vi "Pelletron_Controller.vi"() -> ()   [LabVIEW 2012, in "AccelNET.lvlib" / "Control_VIs.lvlib"]
uses:
  Control_VIs.lvlib
  Component_Power_Indicator.ctl
  Interlocks.ctl
  Bypass_Indicator.ctl
  Parameters_Indicator.ctl
  Parameters_Control.ctl
  Conditioning.ctl
  Component_Power_Control.ctl
  Bypass_Control.ctl
  Database2.0/Public API/PelletronLabview.ctl
  <vilib>/Utility/miscctls.llb/LVPointTypeDef.ctl
  TCPinfo.vi
  TCP.lvclass
  Global_Variables.lvlib
  Useful_SubVIs.lvlib
  Useful_Controls.lvlib
panel:
  out "uA/kV":dbl
  in  "Post to database?":bool=TRUE
  out "Connection Status":bool
  out "Bypass Turn Off":dbl format="%<%H:%M:%S>t"
  in  "Synch":bool
  out "Interlock Status":T1
  in  "Y Log Scale?":bool
  in  "X Maximum":dbl max=0.0 step=30.0 format="%<%H:%M:%S>t"
  in  "X Autoscale":bool=TRUE
  in  "X Minimum":dbl max=0.0 step=30.0 format="%<%H:%M:%S>t"
  in  "Y Autoscale":bool=TRUE
  in  "Y Maximum":dbl
  in  "Y Minimum":dbl
  out "Start Time":dbl format="%<%m/%d/%Y  -  %H:%M:%S>T"
  in  "Clear":bool
  out "XY Graph":cluster{dbl[], dbl[]}(graph)
  in  "Plotter Selector":u16(ring) items=["High Voltage", "High Voltage PS", "Chain Current", "Column Current", "Lost Charge", "Radiation", "Pressure", "HV Control Difference"]
  out "Stop Checking for Sparks Start":dbl
  in  "Stop Condition":bool
  in  "Spark Counter Reset":bool
  in  "Update Parameters":bool
  in  "Param Controls":T2 {"Control Reference\nVoltage (MV)" min=0.3 max=3.0 step=0.1; "High Voltage\nPS Setting (kV)" min=0.0 max=18.0 step=0.2; "Spark\nLimit" min=0.0 max=10.0 step=1.0}
  out "Parameters":T3 {"High\nVoltage (MV)" format="%#.4g"; "Control Reference\nVoltage (MV)" format="%#.4g"; "+ High Voltage\nPS (kV)" format="%#.4g"; "- High Voltage\nPS (kV)" format="%#.4g"; "HV Control\nDifference (kV)" format="%#.4g"; "High Voltage\nPS Setting (kV)" format="%#.4g"; "Chain\nCurrent (uA)" format="%#.4g"; "Column\nCurrent (uA)" format="%#.4g"; "Spark\nLimit" format="%#.0g"; "Spark\nCount" format="%#.0g"; "Lost Charge (uA)" scale=-10.0..10.0; "Spark\nThreshold (MV)" format="%#.4g"; "Radiation (mRad/hr)" step=3.978696e-316 scale=0.02..200.0 scale format="%#.4f"; "Vacuum (Torr)" scale=1e-09..0.001 scale format="%#_6e"}
  out "Warning!":bool
  in  "Reset":bool
  out "Rad. Avg.":dbl(slide) scale=0.02..200.0 scale format="%.0e"
  out "Stopped":bool
  out "Spark\nCounter":i64
  in  "Spark Limit":i64=2
  in  "Emergency Stop":bool
  out "Accelnet Write Errors":errorcluster
  in  "Clear Errors":bool
  out "Accelnet Read Errors":errorcluster
  in  "stop":bool
  out "Condition\nStart Time":dbl format="%<%H:%M:%S>T"
  in  "Conditioning":T4
  in  "Bypass Control":T5
  in  "Update Bypass":bool
  out "Pelletron Bypass":T6
  in  "Component Power Control":T7
  in  "Update On/off":bool
  out "Component\nPower":T8
  # "Instructions:\n\n1) Make sure TCP Control is on and the connection is open.  This is true if you can see TCP information on the top where it says IP Address.\n\n2) Turn on the Pelletron Controller\n\n3) Check to see that the Blower and Ion Gauge Filament is on\n\n4) Check all interlocks are lighte and all bypasses are not.\n\n5) Controls are separate from readings.  Pressing the update button in each respective section sends the commands to the Accelnet system.\n\n6) If the Stopped light is on, then the system will lock out all Pelletron controls and shut off the system until the Reset button is pressed.\n\n7) When finished, stop program with Stop button (make sure Pelletron is off)."
  # "Pelletron Startup Sequence:\n1.  Turn on HV Power Supply\n2. Check +High Voltage PS under parameters to be 1 kV if not change it using the High Voltage PS Setting\n3. Turn on Chain PS\n4. Turn on Chain\n5. Condition Pelletron using auto conditioner or manually using High Voltage PS Setting under Parameter Control\n6.  Check Control Reference Voltage under Parameters to be desired voltage and change it if it is not\n7.  Open Beamline Gate Valve\n8.  Turn on Control Mode\n9.  Turn on Rotating Shaft\n10. Operate Pelletron source through Andrew's Box"
  # "Pelletron Shutdown Sequence:\n1.  Make sure Andrew's box is turned down and off\n2.  Turn off Rotating Shaft\n3.  Check High Voltage PS Setting to be close to + High Voltage PS, if not set it to ~0.2kV above the current setting\n4.  Turn off Control Mode\n5. Close Beamline Gatevalve\n         a.  If you are leaving the pelletron on but the accelerator off, stop here.\n6.  Set Voltage to 1 kv using HighVoltage PS Setting\n7.  Turn off Chain\n8.  Turn off Chain PS and HV Power Supply\n9.  Stop the program."
  # "Interlocks"
  # "Pelletron Plotter"
  # "Parameter Control"
  # "Parameters"
  # "LabVIEW Interlocks"
  # "Pelletron\n   Stop"
  # "Conditioning"
  # "Bypass"
  # "Component On/Off"
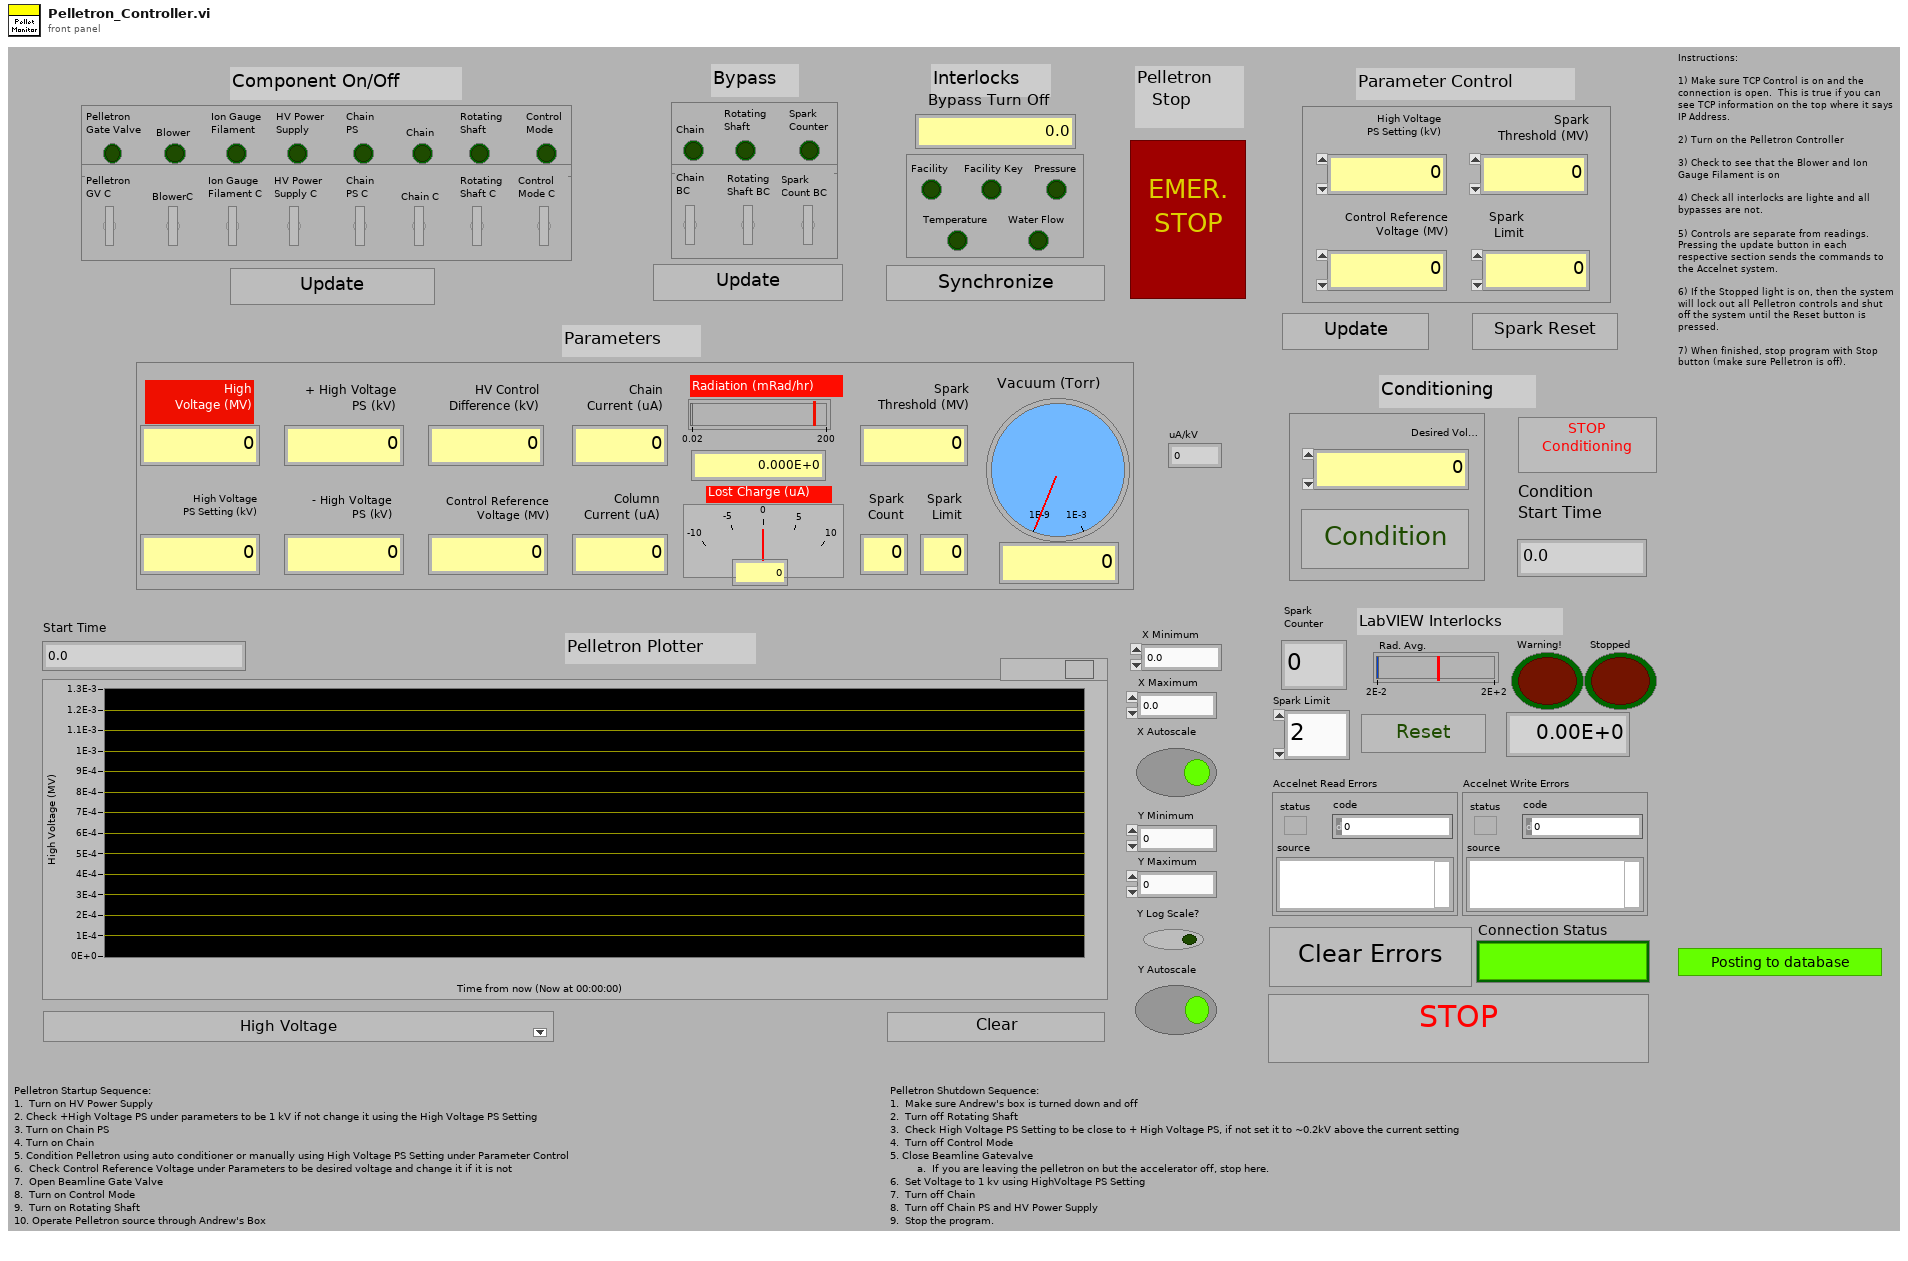
[diagram p1: front panel]
types:
  T1 = typedef "AccelNET.lvlib/Useful_Controls.lvlib/Interlocks.ctl" = cluster{"Facility":bool, "Facility Key":bool, "Water Flow":bool, "Pressure":bool, "Temperature":bool}
  T2 = typedef "AccelNET.lvlib/Useful_Controls.lvlib/Parameters_Control.ctl" = cluster{"Spark\nThreshold (MV)":dbl, "Spark\nLimit":dbl, "High Voltage\nPS Setting (kV)":dbl, "Control Reference\nVoltage (MV)":dbl}
  T3 = typedef "AccelNET.lvlib/Useful_Controls.lvlib/Parameters_Indicator.ctl" = cluster{"Vacuum (Torr)":dbl, "Radiation (mRad/hr)":dbl, "Spark\nThreshold (MV)":dbl, "Lost Charge (uA)":dbl, "Spark\nCount":dbl, "Spark\nLimit":dbl, "Column\nCurrent (uA)":dbl, "Chain\nCurrent (uA)":dbl, "High Voltage\nPS Setting (kV)":dbl, "HV Control\nDifference (kV)":dbl, "- High Voltage\nPS (kV)":dbl, "+ High Voltage\nPS (kV)":dbl, "Control Reference\nVoltage (MV)":dbl, "High\nVoltage (MV)":dbl}
  T4 = typedef "AccelNET.lvlib/Useful_Controls.lvlib/Conditioning.ctl" = cluster{"Desired Voltage (MV)":dbl, "Conditioning?":bool}
  T5 = typedef "AccelNET.lvlib/Useful_Controls.lvlib/Bypass_Control.ctl" = cluster{"Chain\nBC":bool, "Rotating\nShaft BC":bool, "Spark\nCount BC":bool}
  T6 = typedef "AccelNET.lvlib/Useful_Controls.lvlib/Bypass_Indicator.ctl" = cluster{"Chain":bool, "Rotating\nShaft":bool, "Spark\nCounter":bool}
  T7 = typedef "AccelNET.lvlib/Useful_Controls.lvlib/Component_Power_Control.ctl" = cluster{"Pelletron\nGV C":bool, "BlowerC":bool, "Chain C":bool, "Rotating\nShaft C":bool, "HV Power\nSupply C":bool, "Ion Gauge\nFilament C":bool, "Control\nMode C":bool, "Chain\nPS C":bool}
  T8 = typedef "AccelNET.lvlib/Useful_Controls.lvlib/Component_Power_Indicator.ctl" = cluster{"Pelletron\nGate Valve":bool, "Blower":bool, "Chain":bool, "Rotating\nShaft":bool, "HV Power\nSupply":bool, "Ion Gauge\nFilament":bool, "Control\nMode":bool, "Chain\nPS":bool}
  T9 = typedef "LVPointTypeDef.ctl" = cluster{"Horizontal":i16, "Vertical":i16}
  T10 = typedef "PelletronLabview.ctl" = cluster{"Timestamp":timestamp, "High Voltage":sgl, "+ High Voltage Supply":dbl, "- High Voltage Supply":dbl, "HV Control Difference":dbl, "Vacuum Pressure":sgl, "Radiation":dbl, "Column Current":sgl, "Lost Charge":dbl, "Chain Current":sgl, "Control High Voltage":dbl}
  T11 = cluster{"Time":dbl, "High Voltage":dbl, "High VoltagePS":dbl, "Chain Current":dbl, "Column Current":dbl, "Lost Charge":dbl, "Radiation":dbl, "Pressure":dbl, "HV Control Difference":dbl}[]
  T12 = cluster{"Spark\nThreshold (MV)":dbl, "Spark\nLimit":dbl, "High Voltage\nPS Setting (kV)":dbl, "Control Reference\nVoltage (MV)":dbl}
  T13 = enum8{"Enabled", "Disabled", "Disabled and Grayed Out"}
  T14 = cluster{"Time":dbl, "High Voltage":dbl, "High VoltagePS":dbl, "Chain Current":dbl, "Column Current":dbl, "Lost Charge":dbl, "Radiation":dbl, "Pressure":dbl, "HV Control Difference":dbl}
  T15 = cluster{"High\nVoltage (MV)":dbl, "Vacuum (Torr)":dbl, "Lost Charge (uA)":dbl, "+ High Voltage\nPS (kV)":dbl}
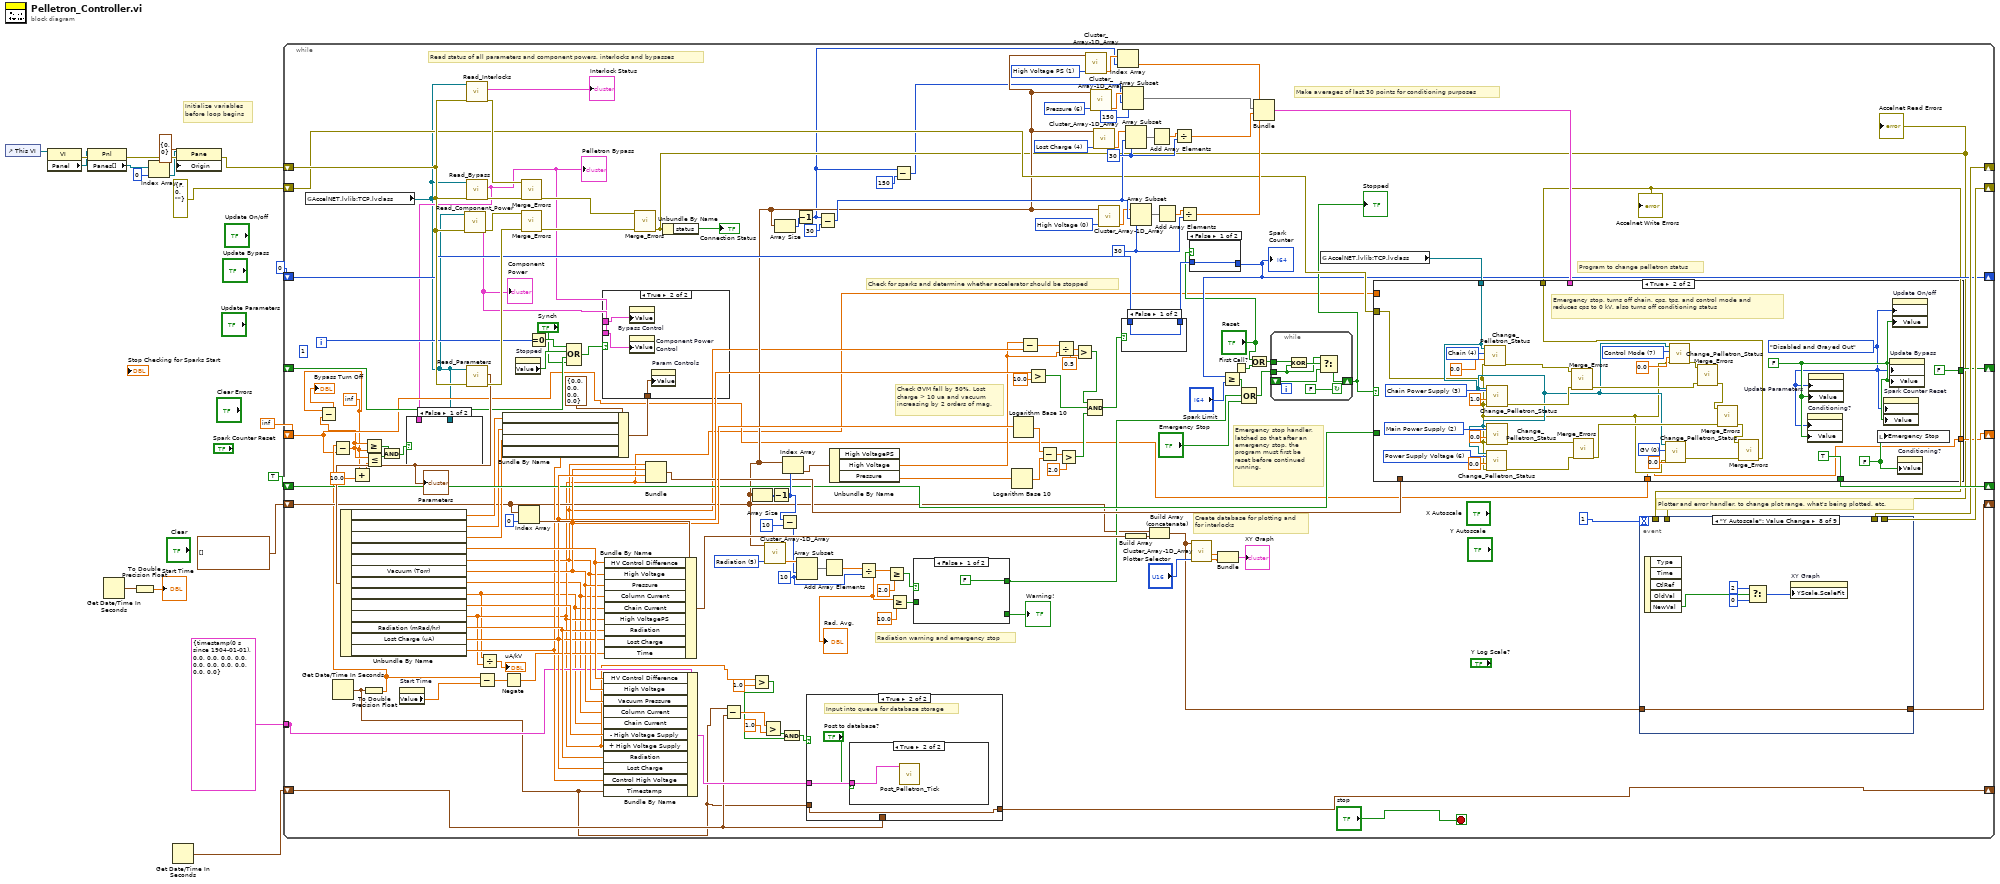
[diagram p0: block diagram]
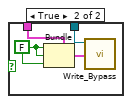
[diagram p4: hidden frame]
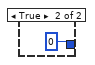
[diagram p5: hidden frame]
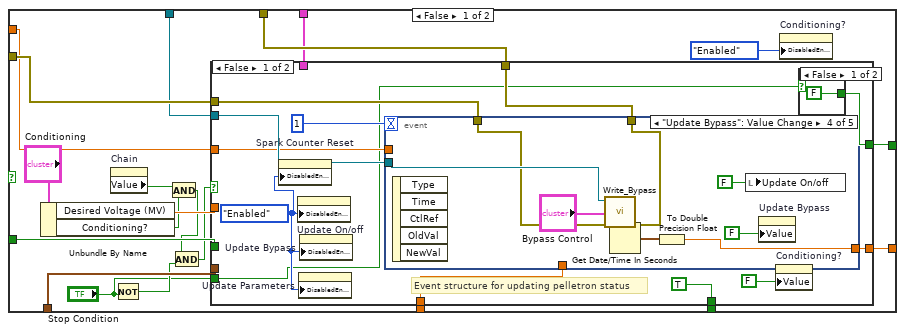
[diagram p7: hidden frame]
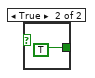
[diagram p8: hidden frame]
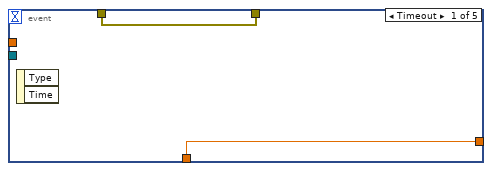
[diagram p9: hidden frame]
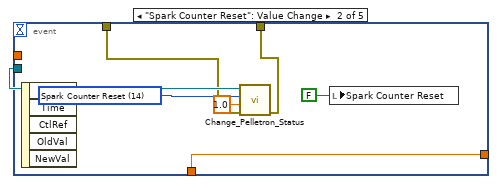
[diagram p10: hidden frame]
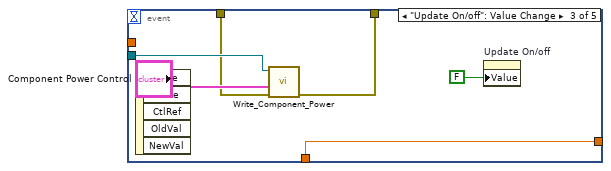
[diagram p11: hidden frame]
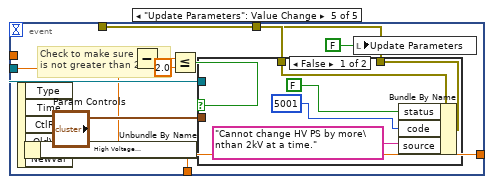
[diagram p12: hidden frame]
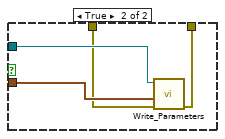
[diagram p13: hidden frame]
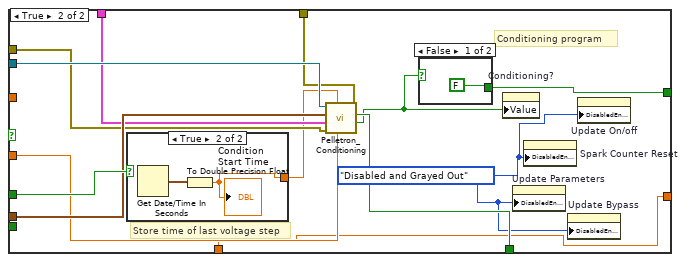
[diagram p14: hidden frame]
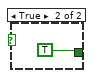
[diagram p15: hidden frame]
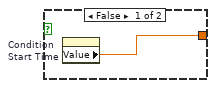
[diagram p16: hidden frame]
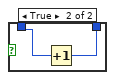
[diagram p17: hidden frame]
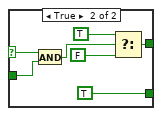
[diagram p18: hidden frame]
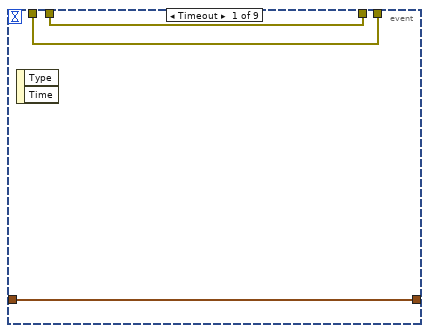
[diagram p19: hidden frame]
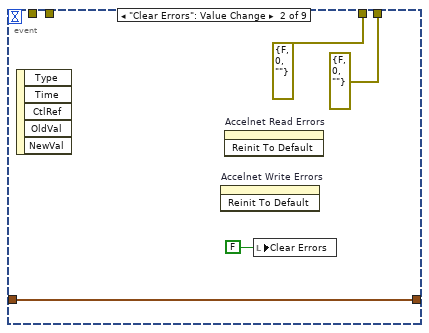
[diagram p20: hidden frame]
diagram:
  # "Initialize variables\nbefore loop begins"
  n1 = control-ref of="This VI"() -> (w9:refnum<vi>)
  n2 = property class="VI"(reference=w9) -> (error out=w8:errorcluster, "Panel"=w7:refnum<vi>)  [unwired: 1 in, 1 out]
  n3 = property class="Pnl"(reference=w7, error in=w8) -> (error out=w6:errorcluster, "Panes[]"=w5:refnum<vi>[])  [unwired: 1 out]
  n4 = Get Date/Time In Seconds() -> (seconds since 1Jan1904=w17:timestamp)
  n5 = To Double Precision Float(number=w17) -> (double precision float=→"Start Time":dbl)
  n6 = Index Array(array=w5, index=0) -> (element=w3:refnum<vi>)
  n7 = Get Date/Time In Seconds() -> (seconds since 1Jan1904=w10:timestamp)
  n8 = property class="Pane"(reference=w3, error in=w6, "Origin"=T9 {"Horizontal"=0, "Vertical"=0}) -> (error out=w1:errorcluster)  [unwired: 1 out]
  n9 = while {
    shift-right: [w98] -> _
    shift-left: w1 -> [w169]
    shift-right: [w154] -> _
    shift-left: T11 [] -> [w82]
    shift-right: [w79] -> _
    shift-left: i64 0 -> [w129]
    shift-right: [w97] -> _
    shift-left: errorcluster {"status"=FALSE, "code"=0, "source"=""} ("error out") -> [w87]
    shift-right: [w102] -> _
    shift-left: TRUE -> [w103]
    shift-right: [w56] -> _
    shift-left: _ -> [w55]
    shift-right: [w53] -> _
    shift-left: inf -> [w51]
    tunnel: [w33] -> _
    tunnel: T10 {"Timestamp"=timestamp(0 s since 1904-01-01), "High Voltage"=0.0, "+ High Voltage Supply"=0.0, "- High Voltage Supply"=0.0, "HV Control Difference"=0.0, "Vacuum Pressure"=0.0, "Radiation"=0.0, "Column Current"=0.0, "Lost Charge"=0.0, "Chain Current"=0.0, "Control High Voltage"=0.0} ("Cluster") -> [w33]
    shift-right: [w31] -> _
    shift-left: w10 -> [w28]
    i -> [w96]
    stop <- "stop" stop-if-true
    w38 = inf ("y")
    (unwired) 1
    w105 = u16 1 items=["High Voltage", "High Voltage PS", "Chain Current", "Column Current", "Lost Charge", "Radiation", "Pressure", "HV Control Difference"] ("Plotter Selector")
    w114 = u16 6 items=["High Voltage", "High Voltage PS", "Chain Current", "Column Current", "Lost Charge", "Radiation", "Pressure", "HV Control Difference"] ("Plotter Selector")
    w115 = 30 ("length")
    w118 = u16 4 items=["High Voltage", "High Voltage PS", "Chain Current", "Column Current", "Lost Charge", "Radiation", "Pressure", "HV Control Difference"] ("Plotter Selector")
    w121 = 30 ("length")
    w126 = u16 0 items=["High Voltage", "High Voltage PS", "Chain Current", "Column Current", "Lost Charge", "Radiation", "Pressure", "HV Control Difference"] ("Plotter Selector")
    w125 = 10 ("length")
    w142 = u16 5 items=["High Voltage", "High Voltage PS", "Chain Current", "Column Current", "Lost Charge", "Radiation", "Pressure", "HV Control Difference"] ("Plotter Selector")
    # "Emergency stop handler,\nlatched so that after an\nemergency stop, the \nprogram must first be \nreset before continued\nrunning."
    # "Plotter and error handler, to change plot range, what's being plotted, etc."
    # "Program to change pelletron status"
    # "Make averages of last 30 points for conditioning purposes"
    # "Check GVM fall by 50%, Lost\ncharge > 10 ua and vacuum\nincreasing by 2 orders of mag."
    # "Create database for plotting and\nfor interlocks"
    # "Radiation warning and emergency stop"
    # "Check for sparks and determine whether accelerator should be stopped"
    # "Read status of all parameters and component powers, interlocks and bypasses"
    n10 = global read "TCPinfo.vi" "AccelNET.lvlib:TCP.lvclass"() -> (w47:refnum<class "TCP.lvclass">)
    n11 = Get Date/Time In Seconds() -> (seconds since 1Jan1904=w27:timestamp)
    n12 = Add(x=w38, y=10.0) -> (x+y=w40:dbl)
    n13 = To Double Precision Float(number=w27) -> (double precision float=w52:dbl)
    n14 = Subtract(x=w52, y=w51) -> (x-y=w45:dbl)
    n15 = Subtract(x=w38, y=w45) -> (x-y=→"Bypass Turn Off":dbl)
    n16 = Greater Or Equal?(x=w45, y=w38) -> (x >= y?=w50:bool)
    n17 = Less Or Equal?(x=w45, y=w40) -> (x <= y?=w49:bool)
    n18 = And(x=w50, y=w49) -> (x .and. y?=w41:bool)
    n19 = property on="Start Time" class="DigNum (strict)"() -> ("Value"=w162:dbl)  [unwired: 2 in, 2 out]
    n20 = call "Read_Component_Power.vi"("error in (no error)"=w169, "AccelNET.lvlib:TCP.lvclass"=w47) -> ("Error Out"=w166:errorcluster, "Component Power"=w54:T8)  [unwired: 8 in]
    "Component\nPower" <- w54
    n21 = call "Read_Interlocks.vi"("Error In"=w169, "AccelNET.lvlib:TCP.lvclass"=w47) -> ("Error Out"=w168:errorcluster, "Interlock Status"=→"Interlock Status":T1)  [unwired: 8 in]
    n22 = call "Read_Bypass.vi"("error in (no error)"=w169, "AccelNET.lvlib:TCP.lvclass"=w47) -> ("Error Out"=w167:errorcluster, "Pelletron Bypass"=w48:T6)  [unwired: 8 in]
    "Pelletron Bypass" <- w48
    n23 = case shown="False" w41 {
      tunnel: w48 -> [_ w178]
      tunnel: w47 -> [_ w175]
      frame False {
      }
      frame True {
        w177 = FALSE ("Chain")
        n24 = Bundle(cluster=w178, "Chain"=w177, "Rotating\nShaft"=w177, "Spark\nCounter"=w177) -> (w176:T6)
        n25 = call "Write_Bypass.vi"("AccelNET.lvlib:TCP.lvclass"=w175, "Pelletron Bypass"=w176) -> ()  [unwired: 8 in, 1 out]
      }
    }
    n26 = call "Read_Parameters.vi"("error in (no error)"=w169, "AccelNET.lvlib:TCP.lvclass"=w47) -> ("Error Out"=w165:errorcluster, "Parameters"=w160:T3)  [unwired: 8 in]
    "Parameters" <- w160
    n27 = Unbundle By Name(w160) -> ("Spark\nThreshold (MV)"=w89:dbl, "Spark\nLimit"=w90:dbl, "High Voltage\nPS Setting (kV)"=w91:dbl, "HV Control\nDifference (kV)"=w147:dbl, "High\nVoltage (MV)"=w66:dbl, "Vacuum (Torr)"=w107:dbl, "Column\nCurrent (uA)"=w20:dbl, "Chain\nCurrent (uA)"=w19:dbl, "- High Voltage\nPS (kV)"=w148:dbl, "+ High Voltage\nPS (kV)"=w22:dbl, "Radiation (mRad/hr)"=w146:dbl, "Lost Charge (uA)"=w108:dbl, "Control Reference\nVoltage (MV)"=w92:dbl)
    n28 = Subtract(x=w52, y=w162) -> (x-y=w150:dbl)
    n29 = Divide(x=w19, y=w22) -> (x/y=→"uA/kV":dbl)
    n30 = Bundle By Name(cluster=T12 {"Spark\nThreshold (MV)"=0.0, "Spark\nLimit"=0.0, "High Voltage\nPS Setting (kV)"=0.0, "Control Reference\nVoltage (MV)"=0.0}, "Spark\nThreshold (MV)"=w89, "Spark\nLimit"=w90, "High Voltage\nPS Setting (kV)"=w91, "Control Reference\nVoltage (MV)"=w92) -> (w93:T12)
    n31 = Negate(x=w150) -> (-x=w145:dbl)
    n32 = property on="Stopped" class="Bool (strict)"() -> ("Value"=w63:bool)  [unwired: 2 in, 2 out]
    n33 = Index Array(array=w82, index=0) -> (element=w152:T14)
    n34 = call "Merge_Errors.vi"("Error 2"=w167, "Error 1"=w168) -> ("Error Out"=w164:errorcluster)  [unwired: 9 in]
    n35 = call "Merge_Errors.vi"("Error 2"=w165, "Error 1"=w166) -> ("Error Out"=w163:errorcluster)  [unwired: 9 in]
    n36 = Equal To 0?(x=w96) -> (x = 0?=w62:bool)
    n37 = Compound Arithmetic op=OR(w62, w63, w55, "Synch") -> (w61:bool)
    n38 = case shown="True" w61 {
      tunnel: w54 -> [_ w188]
      tunnel: w48 -> [_ w189]
      tunnel: w93 -> [_ w187]
      frame False {
      }
      frame True {
        n39 = property on="Bypass Control" class="Clust (strict)"("Value"=w189) -> ()  [unwired: 2 in, 2 out]
        n40 = property on="Component Power Control" class="Clust (strict)"("Value"=w188) -> ()  [unwired: 2 in, 2 out]
        n41 = property on="Param Controls" class="Clust (strict)"("Value"=w187) -> ()  [unwired: 2 in, 2 out]
      }
    }
    n42 = Bundle By Name(cluster=w33, "HV Control Difference"=w147, "High Voltage"=w66, "Vacuum Pressure"=w107, "Column Current"=w20, "Chain Current"=w19, "- High Voltage Supply"=w148, "+ High Voltage Supply"=w22, "Radiation"=w146, "Lost Charge"=w108, "Control High Voltage"=w92, "Timestamp"=w27) -> (w32:T10)
    n43 = Bundle By Name(cluster=w152, "HV Control Difference"=w147, "High Voltage"=w66, "Pressure"=w107, "Column Current"=w20, "Chain Current"=w19, "High VoltagePS"=w22, "Radiation"=w146, "Lost Charge"=w108, "Time"=w145) -> (w155:T14)
    n44 = call "Merge_Errors.vi"("Error 2"=w163, "Error 1"=w164) -> ("Error Out"=w43:errorcluster)  [unwired: 9 in]
    "Accelnet Read Errors" <- w43
    n45 = Bundle("High\nVoltage (MV)"=w66, "Vacuum (Torr)"=w107, "Lost Charge (uA)"=w108, "+ High Voltage\nPS (kV)"=w22) -> (w106:T15)  [unwired: 1 in]
    n46 = Unbundle By Name(w43) -> ("status"=→"Connection Status":bool)
    n47 = Subtract(x=w27, y=w28) -> (x-y=w29:dbl)
    n48 = Greater?(x=w22, y=1.0) -> (0:w24:bool)
    n49 = Array Size(array=w82) -> (size(s)=w144:i32)
    n50 = Greater?(x=w29, y=1.0 ("x")) -> (0:w26:bool)
    n51 = call "Cluster_Array-1D_Array.vi"("Plotter Selector"=w142, "Input Cluster"=w82) -> ("Output Data"=w141:dbl[])  [unwired: 8 in, 1 out]
    n52 = Decrement(x=w144) -> (x-1=w140:i32)
    n53 = Array Size(array=w82) -> (size(s)=w120:i32)
    n54 = Subtract(x=w140, y=10) -> (x-y=w124:i32)
    n55 = And(x=w26, y=w24) -> (x .and. y?=w25:bool)
    n56 = Index Array(array=w82, index=w140) -> (element=w143:T14)
    n57 = Decrement(x=w120) -> (x-1=w35:i32)
    n58 = Array Subset(array=w141, index=w124, length=w125) -> (w138:dbl[])
    n59 = case shown="True" w25 {
      tunnel: w32 -> [_ w173]
      tunnel: w28 -> [w170 _]
      tunnel: [w170 w172] -> w31
      tunnel: w27 -> [_ w172]
      frame False {
      }
      frame True {
        # "Input into queue for database storage"
        n60 = case shown="True" "Post to database?" {
          tunnel: w173 -> [_ w174]
          frame False {
          }
          frame True {
            n61 = call "Post_Pelletron_Tick.vi"("Input data"=w174) -> ()  [unwired: 9 in, 1 out]
          }
        }
      }
    }
    n62 = Subtract(x=w35, y=30) -> (x-y=w112:i32)
    n63 = Add Array Elements(numeric array=w138) -> (sum=w137:dbl)
    n64 = Unbundle By Name(w143) -> ("High Voltage"=w65:dbl, "Pressure"=w131:dbl)  [unwired: 1 out]
    n65 = Divide(x=w137, y=w125) -> (x/y=w88:dbl)
    "Rad. Avg." <- w88
    n66 = Greater Or Equal?(x=w88, y=2.0) -> (x >= y?=w134:bool)
    n67 = Greater Or Equal?(x=w88, y=10.0) -> (x >= y?=w133:bool)
    n68 = Subtract(x=w35, y=150) -> (x-y=w34:i32)
    n69 = case shown="False" w134 {
      selector: w134 -> [_ w326]
      tunnel: w133 -> [_ w325]
      tunnel: [w319 w320] -> w100
      tunnel: [w319 TRUE] -> w132
      frame False {
        w319 = FALSE
      }
      frame True {
        n70 = And(x=w326, y=w325) -> (x .and. y?=w323:bool)
        n71 = Select(t=TRUE, s=w323, f=FALSE) -> (s? t:f=w320:bool)
      }
    }
    "Warning!" <- w132
    n72 = Logarithm Base 10(1:w131) -> (0:w73:dbl)
    n73 = Logarithm Base 10(1:w107) -> (0:w74:dbl)
    n74 = Subtract(x=w65, y=w66) -> (x-y=w67:dbl)
    n75 = Greater?(x=w108, y=10.0) -> (0:w69:bool)
    n76 = Subtract(x=w74, y=w73) -> (x-y=w72:dbl)
    n77 = Divide(x=w67, y=w65) -> (x/y=w77:dbl)
    n78 = Greater?(x=w72, y=2.0) -> (0:w70:bool)
    n79 = Greater?(x=w77, y=0.5) -> (0:w68:bool)
    n80 = call "Cluster_Array-1D_Array.vi"("Plotter Selector"=w105, "Input Cluster"=w82) -> ("Output Data"=w57:dbl[])  [unwired: 8 in, 1 out]
    n81 = Compound Arithmetic op=AND(w68, w69, w70) -> (w130:bool)
    n82 = call "Cluster_Array-1D_Array.vi"("Plotter Selector"=w114, "Input Cluster"=w82) -> ("Output Data"=w58:dbl[])  [unwired: 8 in, 1 out]
    n83 = call "Cluster_Array-1D_Array.vi"("Plotter Selector"=w118, "Input Cluster"=w82) -> ("Output Data"=w59:dbl[])  [unwired: 8 in, 1 out]
    n84 = call "Cluster_Array-1D_Array.vi"("Plotter Selector"=w126, "Input Cluster"=w82) -> ("Output Data"=w60:dbl[])  [unwired: 8 in, 1 out]
    n85 = Index Array(array=w57, index=w35) -> (element=w104:dbl)
    n86 = case shown="False" w130 {
      tunnel: w129 -> [w316 w318]
      tunnel: [w316 w317] -> w80
      frame False {
      }
      frame True {
        n87 = Increment(x=w318) -> (x+1=w317:i64)
      }
    }
    n88 = Array Subset(array=w58, index=w34, length=150) -> (w81:dbl[])
    n89 = Array Subset(array=w59, index=w112, length=w115) -> (w117:dbl[])
    n90 = Build Array(w155) -> (w149:T11)
    n91 = Array Subset(array=w60, index=w112, length=w121) -> (w123:dbl[])
    n92 = Build Array (concatenate)(w82, w149) -> (w151:T11)
    n93 = Add Array Elements(numeric array=w117) -> (sum=w116:dbl)
    n94 = Add Array Elements(numeric array=w123) -> (sum=w122:dbl)
    n95 = Divide(x=w116, y=w115) -> (x/y=w111:dbl)
    n96 = Divide(x=w122, y=w121) -> (x/y=w110:dbl)
    n97 = case shown="False" "Reset" {
      tunnel: [w179 i64 0] -> w79
      tunnel: w80 -> [w179 _]
      frame False {
      }
      frame True {
      }
    }
    "Spark\nCounter" <- w79
    n98 = call "Cluster_Array-1D_Array.vi"("Plotter Selector"="Plotter Selector", "Input Cluster"=w151) -> ("Output Data"=w158:dbl[], "Time"=w156:dbl[])  [unwired: 8 in]
    n99 = Bundle("Time"=w156, "Output Data"=w158) -> (→"XY Graph":cluster{"Time":dbl[], "Output Data":dbl[]})  [unwired: 1 in]
    n100 = Greater Or Equal?(x=w79, y="Spark Limit") -> (x >= y?=w101:bool)
    n101 = First Call?() -> (First Call?: T/F=w84:bool)
    n102 = Compound Arithmetic op=OR(w101, w100, "Emergency Stop") -> (w86:bool)
    n103 = Or(x="Reset", y=w84) -> (x .or. y?=w83:bool)
    n104 = Bundle("Vacuum (Torr)"=w104, w81, w111, w110) -> (w109:cluster{"Vacuum (Torr)":dbl, dbl[], dbl, dbl})  [unwired: 1 in]
    n105 = while {
      shift-right: [w183] -> w85
      shift-left: _ -> [w181]
      tunnel: w86 -> [w184]
      tunnel: w83 -> [w182]
      stop <- FALSE continue-if-true
      n106 = Exclusive Or(1:w184, 2:w182) -> (0:w185:bool)
      n107 = Select(t=w184, s=w185, f=w181) -> (s? t:f=w183:bool)
    }
    "Stopped" <- w85
    n108 = global read "TCPinfo.vi" "AccelNET.lvlib:TCP.lvclass"() -> (w127:refnum<class "TCP.lvclass">)
    n109 = case shown="True" w85 {
      tunnel: w87 -> [w207 w292]
      tunnel: [w206 w289] -> w64
      tunnel: w127 -> [w205 w294]
      tunnel: w109 -> [w204 _]
      tunnel: w106 -> [w203 _]
      tunnel: w103 -> [w202 _]
      tunnel: [w201 TRUE] -> w102
      tunnel: w22 -> [w200 _]
      tunnel: [w194 FALSE ("Value")] -> w56
      tunnel: [w191 w285] -> w53
      tunnel: w51 -> [w190 w285]
      frame False {
        n110 = Unbundle By Name("Conditioning") -> ("Desired Voltage (MV)"=w208:dbl, "Conditioning?"=w199:bool)
        n111 = property on="Chain" class="Bool (strict)"() -> ("Value"=w198:bool)  [unwired: 2 in, 2 out]
        n112 = Not(x="Stop Condition") -> (.not. x?=w196:bool)
        n113 = And(x=w198, y=w199) -> (x .and. y?=w197:bool)
        n114 = And(x=w197, y=w196) -> (x .and. y?=w193:bool)
        n115 = case shown="False" w193 {
          tunnel: w208 -> [_ w273]
          tunnel: w207 -> [w218 w275]
          tunnel: [w217 w274] -> w206
          tunnel: w205 -> [w219 w278]
          tunnel: w204 -> [_ w276]
          tunnel: w203 -> [_ w277]
          tunnel: w202 -> [_ w279]
          tunnel: [TRUE w271] -> w201
          tunnel: w200 -> [w216 _]
          tunnel: [w213 w268] -> w194
          tunnel: "Stop Condition" -> [w212 _]
          tunnel: [w211 w267] -> w191
          tunnel: w190 -> [w210 w267]
          frame False {
            w214 = T13."Enabled" ("Disabled")
            # "Event structure for updating pelletron status"
            n116 = property on="Spark Counter Reset" class="Bool (strict)"("DisabledEnum"=w214) -> ()  [unwired: 2 in, 2 out]
            n117 = property on="Update On/off" class="Bool (strict)"("DisabledEnum"=w214) -> ()  [unwired: 2 in, 2 out]
            n118 = property on="Update Parameters" class="Bool (strict)"("DisabledEnum"=w214) -> ()  [unwired: 2 in, 2 out]
            n119 = property on="Update Bypass" class="Bool (strict)"("DisabledEnum"=w214) -> ()  [unwired: 2 in, 2 out]
            n120 = event shown="[3] \"Update Bypass\": Value Change" {
              selector: _ -> [_ _ _ _ _]
              dyn-events: _ -> [_ _ _ _ _]
              timeout: 1 -> [_ _ _ _ _]
              tunnel: w219 -> [_ w232 w237 w246 w257]
              tunnel: w218 -> [w225 w230 w236 w245 w256]
              tunnel: [w225 w228 w235 w244 w255] -> w217
              tunnel: w216 -> [_ _ _ _ w253]
              tunnel: [w224 w226 w233 w241 w247] -> w211
              tunnel: w210 -> [w224 w226 w233 _ w247]
              event Timeout {
                n121 = event-data() -> ()  [unwired: 1 in, 2 out]
              }
              event "Spark Counter Reset": Value Change {
                w231 = u16 14 items=["GV", "Blower", "Main Power Supply", "Chain Power Supply", "Chain", "Rotating Shaft", "Power Supply Voltage", "Control Mode", "Control Mode Reference", "Chain Bypass", "Rotating Shaft Bypass", "Spark Counter", "Spark Limit", "Threshold", "Spark Counter Reset", "Ion Filament"] ("Write Selector")
                n122 = event-data() -> ()  [unwired: 1 in, 5 out]
                n123 = call "Change_Pelletron_Status.vi"("error in (no error)"=w230, "Write Value"=1.0, "Write Selector"=w231, "AccelNET.lvlib:TCP.lvclass"=w232) -> ("error out"=w228:errorcluster)  [unwired: 7 in]
                n124 = local write "Spark Counter Reset"(FALSE ("Spark Counter Reset")) -> ()
              }
              event "Update On/off": Value Change {
                n125 = event-data() -> ()  [unwired: 1 in, 5 out]
                n126 = call "Write_Component_Power.vi"("AccelNET.lvlib:TCP.lvclass"=w237, "Component Power"="Component Power Control", "error in (no error)"=w236) -> ("Error Out"=w235:errorcluster)  [unwired: 7 in]
                n127 = property on="Update On/off" class="Bool (strict)"("Value"=FALSE ("Update On/off")) -> ()  [unwired: 2 in, 2 out]
              }
              event "Update Bypass": Value Change {
                n128 = event-data() -> ()  [unwired: 1 in, 5 out]
                n129 = call "Write_Bypass.vi"("AccelNET.lvlib:TCP.lvclass"=w246, "Pelletron Bypass"="Bypass Control", "error in (no error)"=w245) -> ("Error Out"=w244:errorcluster)  [unwired: 7 in]
                n130 = Get Date/Time In Seconds() -> (seconds since 1Jan1904=w239:timestamp)
                n131 = To Double Precision Float(number=w239) -> (double precision float=w241:dbl)
                n132 = local write "Update On/off"(FALSE ("Update On/off")) -> ()
                n133 = property on="Update Bypass" class="Bool (strict)"("Value"=FALSE ("Update Bypass")) -> ()  [unwired: 2 in, 2 out]
              }
              event "Update Parameters": Value Change {
                # "Check to make sure step\nis not greater than 2kV"
                n134 = event-data() -> ()  [unwired: 1 in, 5 out]
                n135 = Unbundle By Name("Param Controls") -> ("High Voltage\nPS Setting (kV)"=w252:dbl)
                n136 = Subtract(x=w252, y=w253) -> (x-y=w251:dbl)
                n137 = Less Or Equal?(x=w251, y=2.0) -> (x <= y?=w249:bool)
                n138 = case shown="False" w249 {
                  tunnel: "Param Controls" -> [_ w266]
                  tunnel: w257 -> [_ w265]
                  tunnel: w256 -> [w262 w264]
                  tunnel: [w258 w263] -> w255
                  frame False {
                    n139 = Bundle By Name(cluster=w262, "status"=FALSE, "code"=5001, "source"="Cannot change HV PS by more\nthan 2kV at a time.") -> (w258:errorcluster)
                  }
                  frame True {
                    n140 = call "Write_Parameters.vi"("error in (no error)"=w264, "Param Controls"=w266, "AccelNET.lvlib:TCP.lvclass"=w265) -> ("Error Out"=w263:errorcluster)  [unwired: 8 in]
                  }
                }
                n141 = local write "Update Parameters"(FALSE ("Update Parameters")) -> ()
              }
            }
            n142 = property on="Conditioning?" class="Bool (strict)"("Value"=FALSE) -> ()  [unwired: 2 in, 2 out]
            n143 = case shown="False" w212 {
              tunnel: [FALSE TRUE] -> w213
              frame False {
              }
              frame True {
              }
            }
          }
          frame True {
            w270 = T13."Disabled and Grayed Out" ("Disabled")
            # "Store time of last voltage step"
            # "Conditioning program"
            n144 = case shown="True" w279 {
              tunnel: [w282 w283] -> w272
              frame False {
                n145 = property on="Condition\nStart Time" class="DigNum (strict)"() -> ("Value"=w282:dbl)  [unwired: 2 in, 2 out]
              }
              frame True {
                n146 = Get Date/Time In Seconds() -> (seconds since 1Jan1904=w284:timestamp)
                n147 = To Double Precision Float(number=w284) -> (double precision float=w283:dbl)
                "Condition\nStart Time" <- w283
              }
            }
            n148 = call "Pelletron_Conditioning.vi"("Desired Voltage (MV)"=w273, "Condition Start time"=w272, "error in (no error)"=w275, "Input Old Cluster"=w276, "Input New Cluster"=w277, "AccelNET.lvlib:TCP.lvclass"=w278) -> ("Error Out"=w274:errorcluster, "Conditioning?"=w269:bool, "Step Up Voltage?"=w271:bool)  [unwired: 3 in]
            n149 = case shown="False" w269 {
              tunnel: [FALSE TRUE] -> w268
              frame False {
              }
              frame True {
              }
            }
            n150 = property on="Conditioning?" class="Bool (strict)"("Value"=w269) -> ()  [unwired: 2 in, 2 out]
            n151 = property on="Update Parameters" class="Bool (strict)"("DisabledEnum"=w270) -> ()  [unwired: 2 in, 2 out]
            n152 = property on="Spark Counter Reset" class="Bool (strict)"("DisabledEnum"=w270) -> ()  [unwired: 2 in, 2 out]
            n153 = property on="Update Bypass" class="Bool (strict)"("DisabledEnum"=w270) -> ()  [unwired: 2 in, 2 out]
            n154 = property on="Update On/off" class="Bool (strict)"("DisabledEnum"=w270) -> ()  [unwired: 2 in, 2 out]
          }
        }
        n155 = property on="Conditioning?" class="Bool (strict)"("DisabledEnum"=T13."Enabled" ("Disabled")) -> ()  [unwired: 2 in, 2 out]
      }
      frame True {
        w288 = FALSE ("Update Parameters")
        w287 = T13."Disabled and Grayed Out" ("Disabled")
        w295 = u16 0 items=["GV", "Blower", "Main Power Supply", "Chain Power Supply", "Chain", "Rotating Shaft", "Power Supply Voltage", "Control Mode", "Control Mode Reference", "Chain Bypass", "Rotating Shaft Bypass", "Spark Counter", "Spark Limit", "Threshold", "Spark Counter Reset", "Ion Filament"] ("Write Selector")
        w296 = FALSE ("Value")
        w305 = u16 7 items=["GV", "Blower", "Main Power Supply", "Chain Power Supply", "Chain", "Rotating Shaft", "Power Supply Voltage", "Control Mode", "Control Mode Reference", "Chain Bypass", "Rotating Shaft Bypass", "Spark Counter", "Spark Limit", "Threshold", "Spark Counter Reset", "Ion Filament"] ("Write Selector")
        w306 = u16 6 items=["GV", "Blower", "Main Power Supply", "Chain Power Supply", "Chain", "Rotating Shaft", "Power Supply Voltage", "Control Mode", "Control Mode Reference", "Chain Bypass", "Rotating Shaft Bypass", "Spark Counter", "Spark Limit", "Threshold", "Spark Counter Reset", "Ion Filament"] ("Write Selector")
        w308 = u16 2 items=["GV", "Blower", "Main Power Supply", "Chain Power Supply", "Chain", "Rotating Shaft", "Power Supply Voltage", "Control Mode", "Control Mode Reference", "Chain Bypass", "Rotating Shaft Bypass", "Spark Counter", "Spark Limit", "Threshold", "Spark Counter Reset", "Ion Filament"] ("Write Selector")
        w312 = u16 3 items=["GV", "Blower", "Main Power Supply", "Chain Power Supply", "Chain", "Rotating Shaft", "Power Supply Voltage", "Control Mode", "Control Mode Reference", "Chain Bypass", "Rotating Shaft Bypass", "Spark Counter", "Spark Limit", "Threshold", "Spark Counter Reset", "Ion Filament"] ("Write Selector")
        w315 = u16 4 items=["GV", "Blower", "Main Power Supply", "Chain Power Supply", "Chain", "Rotating Shaft", "Power Supply Voltage", "Control Mode", "Control Mode Reference", "Chain Bypass", "Rotating Shaft Bypass", "Spark Counter", "Spark Limit", "Threshold", "Spark Counter Reset", "Ion Filament"] ("Write Selector")
        # "Emergency stop, turns off chain, cps, tps, and control mode and reduces cps to 0 kV, also turns off conditioning status"
        n156 = call "Change_Pelletron_Status.vi"("error in (no error)"=w292, "Write Value"=0.0, "Write Selector"=w315, "AccelNET.lvlib:TCP.lvclass"=w294) -> ("error out"=w311:errorcluster)  [unwired: 7 in]
        n157 = call "Change_Pelletron_Status.vi"("error in (no error)"=w292, "Write Value"=0.0, "Write Selector"=w306, "AccelNET.lvlib:TCP.lvclass"=w294) -> ("error out"=w302:errorcluster)  [unwired: 7 in]
        n158 = call "Change_Pelletron_Status.vi"("error in (no error)"=w292, "Write Value"=1.0, "Write Selector"=w312, "AccelNET.lvlib:TCP.lvclass"=w294) -> ("error out"=w310:errorcluster)  [unwired: 7 in]
        n159 = call "Change_Pelletron_Status.vi"("error in (no error)"=w292, "Write Value"=0.0, "Write Selector"=w308, "AccelNET.lvlib:TCP.lvclass"=w294) -> ("error out"=w303:errorcluster)  [unwired: 7 in]
        n160 = call "Merge_Errors.vi"("Error 2"=w310, "Error 1"=w311) -> ("Error Out"=w300:errorcluster)  [unwired: 9 in]
        n161 = call "Merge_Errors.vi"("Error 2"=w302, "Error 1"=w303) -> ("Error Out"=w299:errorcluster)  [unwired: 9 in]
        n162 = call "Change_Pelletron_Status.vi"("error in (no error)"=w292, "Write Value"=0.0, "Write Selector"=w295, "AccelNET.lvlib:TCP.lvclass"=w294) -> ("error out"=w290:errorcluster)  [unwired: 7 in]
        n163 = call "Change_Pelletron_Status.vi"("error in (no error)"=w292, "Write Value"=0.0, "Write Selector"=w305, "AccelNET.lvlib:TCP.lvclass"=w294) -> ("error out"=w301:errorcluster)  [unwired: 7 in]
        n164 = call "Merge_Errors.vi"("Error 2"=w300, "Error 1"=w301) -> ("Error Out"=w298:errorcluster)  [unwired: 9 in]
        n165 = call "Merge_Errors.vi"("Error 2"=w299, "Error 1"=w298) -> ("Error Out"=w291:errorcluster)  [unwired: 9 in]
        n166 = call "Merge_Errors.vi"("Error 2"=w290, "Error 1"=w291) -> ("Error Out"=w289:errorcluster)  [unwired: 9 in]
        n167 = property on="Conditioning?" class="Bool (strict)"("DisabledEnum"=w287, "Value"=w288) -> ()  [unwired: 2 in, 2 out]
        n168 = property on="Update Parameters" class="Bool (strict)"("DisabledEnum"=w287, "Value"=w288) -> ()  [unwired: 2 in, 2 out]
        n169 = local write "Emergency Stop"(w296) -> ()
        n170 = property on="Spark Counter Reset" class="Bool (strict)"("DisabledEnum"=w287, "Value"=w288) -> ()  [unwired: 2 in, 2 out]
        n171 = property on="Update Bypass" class="Bool (strict)"("DisabledEnum"=w287, "Value"=w288) -> ()  [unwired: 2 in, 2 out]
        n172 = property on="Update On/off" class="Bool (strict)"("DisabledEnum"=w287, "Value"=w288) -> ()  [unwired: 2 in, 2 out]
        n173 = property on="Conditioning?" class="Bool (strict)"("Value"=w296) -> ()  [unwired: 2 in, 2 out]
      }
    }
    "Accelnet Write Errors" <- w64
    n174 = event shown="[7] \"Y Autoscale\": Value Change" {
      selector: _ -> [_ _ _ _ _ _ _ _ _]
      dyn-events: _ -> [_ _ _ _ _ _ _ _ _]
      timeout: 1 -> [_ _ _ _ _ _ _ _ _]
      tunnel: w151 -> [w329 w333 w334 _ w348 w351 w364 w365 w375]
      tunnel: [w329 w333 w334 T11 [] w348 w351 w364 w365 w375] -> w154
      tunnel: w64 -> [w327 _ _ w339 w346 w355 w362 _ w372]
      tunnel: w43 -> [w328 _ _ w340 w347 w356 w363 _ w373]
      tunnel: [w328 errorcluster {"status"=FALSE, "code"=0, "source"=""} ("Error Out") _ w340 w347 w356 w363 _ w373] -> w98
      tunnel: [w327 errorcluster {"status"=FALSE, "code"=0, "source"=""} ("Error Out") _ w339 w346 w355 w362 _ w372] -> w97
      event Timeout {
        n175 = event-data() -> ()  [unwired: 1 in, 2 out]
      }
      event "Clear Errors": Value Change {
        n176 = event-data() -> ()  [unwired: 1 in, 5 out]
        n177 = invoke on="Accelnet Write Errors" class="Clust (strict)" method="Reinit To Default"() -> ()  [unwired: 3 in, 3 out]
        n178 = invoke on="Accelnet Read Errors" class="Clust (strict)" method="Reinit To Default"() -> ()  [unwired: 3 in, 3 out]
        n179 = local write "Clear Errors"(FALSE ("Clear Errors")) -> ()
      }
      event "Y Log Scale?": Value Change {
        n180 = event-data() -> ("NewVal"=w336:bool)  [unwired: 1 in, 4 out]
        n181 = Select(t=u8 1, s=w336, f=u8 0) -> (s? t:f=w337:u8)
        n182 = property on="XY Graph" class="XYGraph (strict)"("YScale.Mapping Mode"=w337) -> ()  [unwired: 2 in, 2 out]
      }
      event "Clear": Value Change {
        n183 = event-data() -> ()  [unwired: 1 in, 5 out]
        n184 = Get Date/Time In Seconds() -> (seconds since 1Jan1904=w343:timestamp)
        n185 = To Double Precision Float(number=w343) -> (double precision float=w342:dbl)
        n186 = local write "Start Time"(w342) -> ()
      }
      event "X Maximum", "X Minimum": Value Change {
        n187 = event-data() -> ()  [unwired: 1 in, 5 out]
        n188 = property on="XY Graph" class="XYGraph (strict)"("XScale.Maximum"="X Maximum", "XScale.Minimum"="X Minimum", "XScale.ScaleFit"=u8 0 ("X Scale.Scale Fit")) -> ()  [unwired: 2 in, 2 out]
        n189 = local write "X Autoscale"(FALSE ("X Autoscale")) -> ()
      }
      event "Y Maximum", "Y Minimum": Value Change {
        n190 = event-data() -> ()  [unwired: 1 in, 5 out]
        n191 = property on="XY Graph" class="XYGraph (strict)"("YScale.Maximum"="Y Maximum", "YScale.Minimum"="Y Minimum", "YScale.ScaleFit"=u8 0 ("Y Scale.Scale Fit")) -> ()  [unwired: 2 in, 2 out]
        n192 = local write "Y Autoscale"(FALSE ("Y Autoscale")) -> ()
      }
      event "X Autoscale": Value Change {
        n193 = event-data() -> ("NewVal"=w359:bool)  [unwired: 1 in, 4 out]
        n194 = Select(t=2, s=w359, f=0) -> (s? t:f=w358:i32)
        n195 = property on="XY Graph" class="XYGraph (strict)"("XScale.ScaleFit"=w358) -> ()  [unwired: 2 in, 2 out]
      }
      event "Y Autoscale": Value Change {
        n196 = event-data() -> ("NewVal"=w369:bool)  [unwired: 1 in, 4 out]
        n197 = Select(t=u8 2, s=w369, f=u8 0) -> (s? t:f=w366:u8)
        n198 = property on="XY Graph" class="XYGraph (strict)"("YScale.ScaleFit"=w366) -> ()  [unwired: 2 in, 2 out]
      }
      event "Plotter Selector": Value Change {
        n199 = event-data() -> ("NewVal"=w376:u16)  [unwired: 1 in, 4 out]
        n200 = case shown="7" w376 {
          tunnel: [0 0 0 0 0 1 1 0] -> w371
          tunnel: ["High Voltage (MV)" "High Voltage Power Supply (kV)" "Chain Current (uA)" "Column Current (uA)" "Lost Charge (uA)" "Radiation (mRad/hr)" "Pressure (torr)" "HV Control Difference (kV)"] -> w374
          frame 0, Default {
          }
          frame 1 {
          }
          frame 2 {
          }
          frame 3 {
          }
          frame 4 {
          }
          frame 5 {
          }
          frame 6 {
          }
          frame 7 {
          }
        }
        n201 = Not Equal To 0?(x=w371) -> (x != 0?=w370:bool)
        n202 = property on="XY Graph" class="XYGraph (strict)"("YScale.Mapping Mode"=w371, "YScale.NameLbl.Text"=w374) -> ()  [unwired: 2 in, 2 out]
        n203 = local write "Y Log Scale?"(w370) -> ()
      }
    }
  }
